vi "RSNRPZ Get ContAv Buffer Info.vi"(7 "Array Size (0)":i32, 8 "error in (no error)":errorcluster, 9 "Info Type (\"\")":string, 10 "Channel (1)":i32=1, 11 "VISA session":refnum<visa-resource-name> caption="VISA resource name") -> (0 "error out":errorcluster, 2 "Info":string, 3 "dup VISA session":refnum<visa-resource-name> caption="VISA resource name")   [LabVIEW 2010]
doc: "This VI returns some important settings for the scalar network analysis.\n\nRemote-control command(s):\nSENS:POW:AVG:BUFF:INFO? <Info Type>"
uses:
  rsnrpz_32.dll
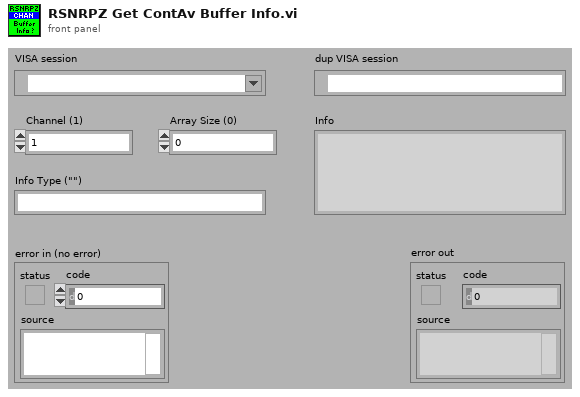
[diagram p1: front panel]
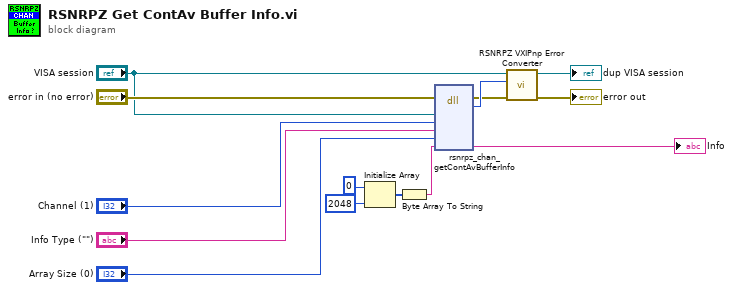
[diagram p0: block diagram]
diagram:
  n1 = Initialize Array(u8 0 ("element"), 2048 ("dimension size")) -> (w8:u8[])
  n2 = Byte Array To String(unsigned byte array=w8) -> (string=w9:string)
  n3 = dll-call lib="rsnrpz_32.dll" fn="rsnrpz_chan_getContAvBufferInfo"(error in="error in (no error)", "Instrument Handle"="VISA session", "Channel"="Channel (1)", "Info Type"="Info Type (\"\")", "Array Size"="Array Size (0)", "Info"=w9) -> (error out=w5:errorcluster, w10:i32, "Info"=→"Info":string)  [unwired: 6 in, 1 out]
  n4 = call <instrlib>:"RSNRPZ VXIPnp Error Converter.vi"("error in"=w5, "VXIPnp error code"=w10, "VISA session"="VISA session") -> ("error out"=→"error out":errorcluster, "dup VISA session"=→"dup VISA session":refnum<visa-resource-name>)  [unwired: 7 in]
